vi "DataLoggerVI.vi"() -> ()   [LabVIEW 2020]
panel:
  in  "VISA resource name":refnum<visa-resource-name>
  in  "Table Control":string[][](table)
  out "Waveform Humidity":dbl(graph)
  out "Waveform Temp":dbl(graph)
  out "Humidity":dbl(knob) scale=0.0..100.0
  out "Temp":dbl(slide) scale=0.0..50.0
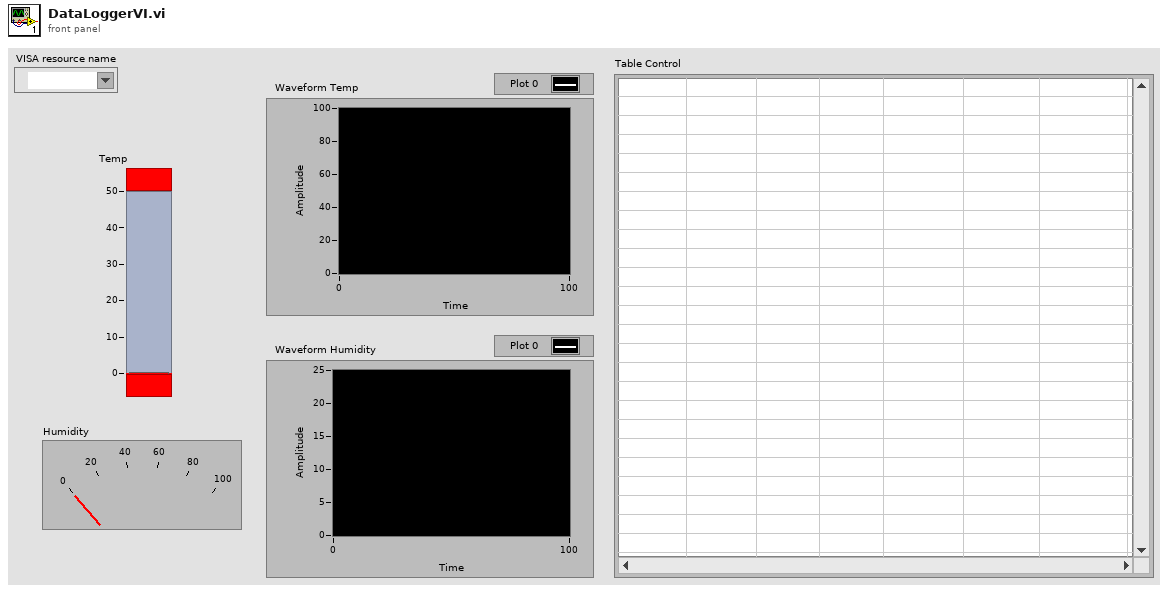
[diagram p1: front panel]
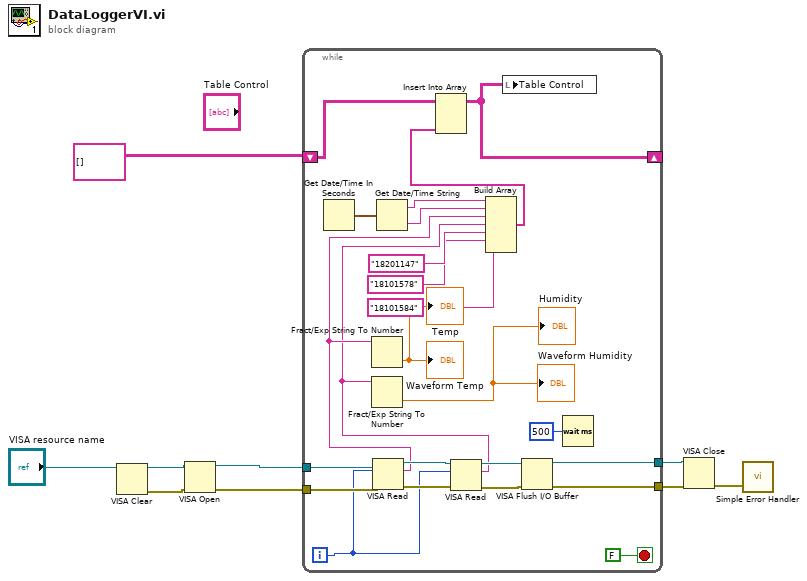
[diagram p0: block diagram]
diagram:
  n1 = VISA Clear(VISA resource name="VISA resource name") -> (VISA resource name out=w9:refnum<visa-resource-name>, error out=w8:errorcluster)  [unwired: 1 in]
  n2 = VISA Open(error in (no error)=w8, VISA resource name=w9) -> (VISA resource name=w6:refnum<visa-resource-name>, error out=w5:errorcluster)  [unwired: 3 in]
  n3 = while {
    tunnel: w6 -> [w33]
    tunnel: w5 -> [w32]
    tunnel: [w27] -> w4
    tunnel: [w26] -> w3
    shift-right: [w22] -> _
    shift-left: string[][] [] -> [w23]
    i -> [w25]
    stop <- FALSE stop-if-true
    n4 = Get Date/Time In Seconds() -> (seconds since 1Jan1904=w19:timestamp)
    n5 = VISA Read(VISA resource name=w33, byte count=w25, error in (no error)=w32) -> (VISA resource name out=w31:refnum<visa-resource-name>, read buffer=w16:string, error out=w30:errorcluster)  [unwired: 1 out]
    n6 = Fract/Exp String To Number(string=w16) -> (number=→"Temp" →"Waveform Temp":dbl)  [unwired: 3 in, 1 out]
    n7 = Get Date/Time String(seconds (now)=w19) -> (date string=w18:string, time string=w17:string)  [unwired: 2 in]
    n8 = VISA Read(VISA resource name=w31, byte count=w25, error in (no error)=w30) -> (VISA resource name out=w29:refnum<visa-resource-name>, read buffer=w15:string, error out=w28:errorcluster)  [unwired: 1 out]
    n9 = Fract/Exp String To Number(string=w15) -> (number=→"Humidity" →"Waveform Humidity":dbl)  [unwired: 3 in, 1 out]
    n10 = Build Array(w18, w17, w16, w15, "18201147" ("element"), "18101578" ("element"), "18101584" ("element")) -> (w13:string[])
    n11 = Insert Into Array(array=w23, new element=w13) -> (w22:string[][])  [unwired: 2 in]
    n12 = local write "Table Control"(w22) -> ()
    n13 = VISA Flush I/O Buffer(VISA resource name=w29, error in (no error)=w28) -> (VISA resource name out=w27:refnum<visa-resource-name>, error out=w26:errorcluster)  [unwired: 1 in]
    n14 = Wait (ms)(milliseconds to wait=u32 500) -> ()  [unwired: 1 out]
  }
  n15 = VISA Close(VISA resource name=w4, error in (no error)=w3) -> (error out=w7:errorcluster)
  n16 = call <vilib>:"Simple Error Handler.vi"("error in (no error)"=w7) -> ()  [unwired: 4 in, 5 out]
